vi "ErrorHandler.vi"(8 "error in (no error)":errorcluster, 11 "queue in":refnum<queue>) -> (0 "error out":errorcluster, 3 "queue out":refnum<queue>)   [LabVIEW 2018, in "MyPlugins.lvlib"]
doc: "Handle an error by enqueueing an \"Error\" message to the front of the queue."
uses:
  MyPlugins/MyPlugins.lvlib
  PublicAPI/Arguments/Messages/clMessage.ctl
  MyPlugins/MyPluginBaseClass/MyPluginsBase.lvclass
panel:
  in  "Message (Error)":string="Error"
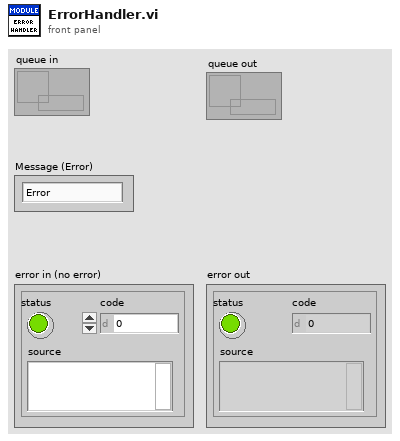
[diagram p1: front panel]
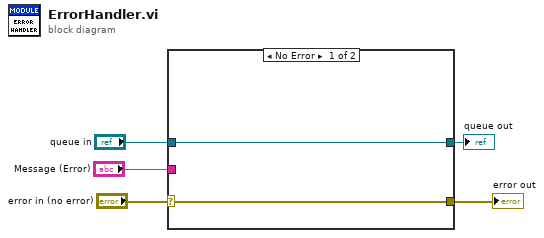
[diagram p0: block diagram]
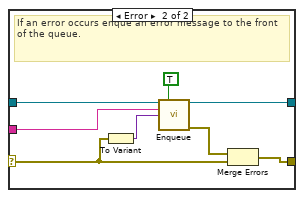
[diagram p2: hidden frame]
diagram:
  n1 = case shown="No Error" "error in (no error)" {
    selector: "error in (no error)" -> [w7 w11]
    tunnel: "Message (Error)" -> [_ w14]
    tunnel: [w6 w12] -> w1
    tunnel: [w7 w10] -> w3
    tunnel: "queue in" -> [w6 w8]
    frame No Error {
    }
    frame Error {
      # "If an error occurs enque an error message to the front of the queue."
      n2 = To Variant(anything=w11) -> (Variant=w15:variant)
      n3 = call "Enqueue.vi"("queue in"=w8, "Priority (F)"=TRUE, "Message"=w14, "Message Data"=w15) -> ("queue out"=w12:refnum<queue>, "error out"=w9:errorcluster)  [unwired: 10 in]
      n4 = Merge Errors(w9, w11) -> (w10:errorcluster)
    }
  }
  "error out" <- w3
  "queue out" <- w1
